vi "Logic.vi"   [LabVIEW 2012]
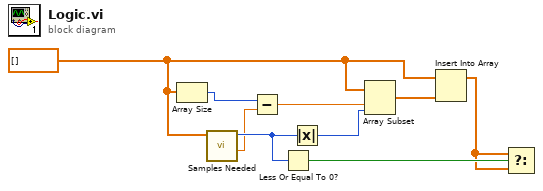
[diagram p0: block diagram]
diagram:
  w1 = dbl[] []
  n1 = Array Size(array=w1) -> (size(s)=w6:i32)
  n2 = call "Samples Needed.vi"("Sample Array"=w1) -> ("Index"=w4:dbl, "Samples Needed"=w8:i32)  [unwired: 9 in]
  n3 = Subtract(x=w6, y=w4) -> (x-y=w5:dbl)
  n4 = Less Or Equal To 0?(x=w8) -> (x <= 0?=w9:bool)
  n5 = Absolute Value(x=w8) -> (abs(x)=w7:i32)
  n6 = Array Subset(array=w1, index=w5, length=w7) -> (w3:dbl[])
  n7 = Insert Into Array(array=w1, new element=w3) -> (w2:dbl[])  [unwired: 1 in]
  n8 = Select(t=w2, s=w9, f=w2) -> ()  [unwired: 1 out]
